vi "DTACQ - Set All Data Sizes.vi"(8 "error in":errorcluster, 10 "Analog In Data Size":T1, 11 "Address":string) -> (0 "error out":errorcluster, 2 "Acknowledged":bool)   [LabVIEW 2017, in "Communications Library.lvlib"]
doc: "Sets the data size for all analog in modules, and the module carrier, to 16 or 32 bits."
uses:
  Communications Library.lvlib
  Typedefs/Data Size--Enum.ctl
  Typedefs/DTACQ Device Type--Enum.ctl
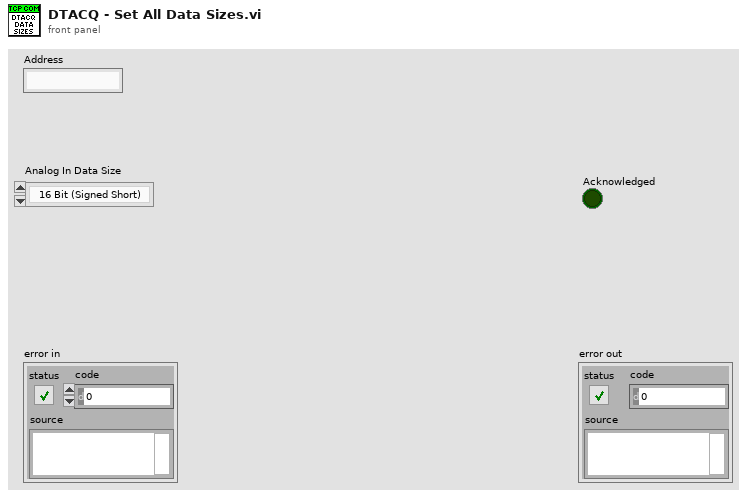
[diagram p1: front panel]
types:
  T1 = typedef "Communications Library.lvlib/Data Size--Enum.ctl" = enum16{"16 Bit (Signed Short)", "32 Bit (Signed Long)"}
  T2 = typedef "Communications Library.lvlib/DTACQ Device Type--Enum.ctl" = enum16{"Carrier", "Analog In Module", "Analog Out Module", "Generic Module"}
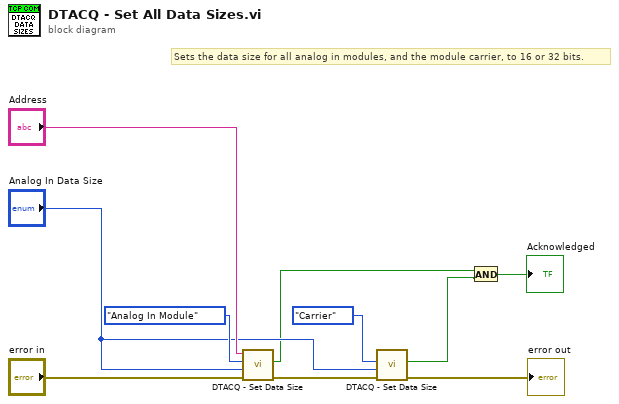
[diagram p0: block diagram]
diagram:
  # "Sets the data size for all analog in modules, and the module carrier, to 16 or 32 bits."
  n1 = call "DTACQ - Set Data Size.vi"("error in"="error in", "Data Size"="Analog In Data Size", "Module Type"=DTACQ_Device_Type--Enum."Analog In Module", "Address"="Address") -> ("error out"=w8:errorcluster, "Acknowledged"=w2:bool)  [unwired: 6 in]
  n2 = call "DTACQ - Set Data Size.vi"("error in"=w8, "Data Size"="Analog In Data Size", "Module Type"=DTACQ_Device_Type--Enum."Carrier") -> ("error out"=→"error out":errorcluster, "Acknowledged"=w3:bool)  [unwired: 7 in]
  n3 = And(x=w2, y=w3) -> (x .and. y?=→"Acknowledged":bool)
